vi "USBPT104Example.vi"() -> ()   [LabVIEW 2017]
uses:
  Instance           1 16Saved   USBPT104 .vi
  UsbPT104.dll
panel:
  out "UnitInfo fields":string[](array[string])=["Driver Version", "USB Version", "Hardware Version", "Variant Info", "Cal Date", "Kernal Driver Version"]
  out "error out":errorcluster={"status"=TRUE, "code"=5037, "source"="UsbPt104GetValue"}
  in  "error in (no error)":errorcluster
  out "UnitInfo":string[](array[string])
  in  "IP Address":string
  in  "Connection":bool
  out "CH4 Value":dbl(slide) max=10000.0 scale=-200.0..800.0
  out "CH3 Value":dbl(slide) max=10000.0 scale=-200.0..800.0
  out "CH2 Value":dbl(slide) max=10000.0 scale=-200.0..800.0
  in  "Update settings":bool
  in  "CH4 Measurement Type":i32(ring) items=["OFF", "PT100", "PT1000", "Resistance to 375 Ohms", "Resistance to 10 kOhms", "Differential to 115 mV", "Differential to 2500 mV", "Single-ended to 115 mV", "Single-ended to 2500 mV"]
  in  "CH4 Number of Wires":i16(ring)=4 items=["2"=2, "3"=3, "4"=4]
  in  "CH3 Measurement Type":i32(ring) items=["OFF", "PT100", "PT1000", "Resistance to 375 Ohms", "Resistance to 10 kOhms", "Differential to 115 mV", "Differential to 2500 mV", "Single-ended to 115 mV", "Single-ended to 2500 mV"]
  in  "CH3 Number of Wires":i16(ring)=4 items=["2"=2, "3"=3, "4"=4]
  in  "CH2 Measurement Type":i32(ring) items=["OFF", "PT100", "PT1000", "Resistance to 375 Ohms", "Resistance to 10 kOhms", "Differential to 115 mV", "Differential to 2500 mV", "Single-ended to 115 mV", "Single-ended to 2500 mV"]
  in  "CH2 Number of Wires":i16(ring)=4 items=["2"=2, "3"=3, "4"=4]
  in  "CH1 Number of Wires":i16(ring)=4 items=["2"=2, "3"=3, "4"=4]
  in  "CH1 Measurement Type":i32(ring)=1 items=["OFF", "PT100", "PT1000", "Resistance to 375 Ohms", "Resistance to 10 kOhms", "Differential to 115 mV", "Differential to 2500 mV", "Single-ended to 115 mV", "Single-ended to 2500 mV"]
  out "CH1 Value":dbl(slide) max=10000.0 scale=-200.0..800.0
  in  "Stop":bool
  # "USB"
  # "Ethernet"
  # "Channel 1"
  # "Channel 2"
  # "Channel 3"
  # "Channel 4"
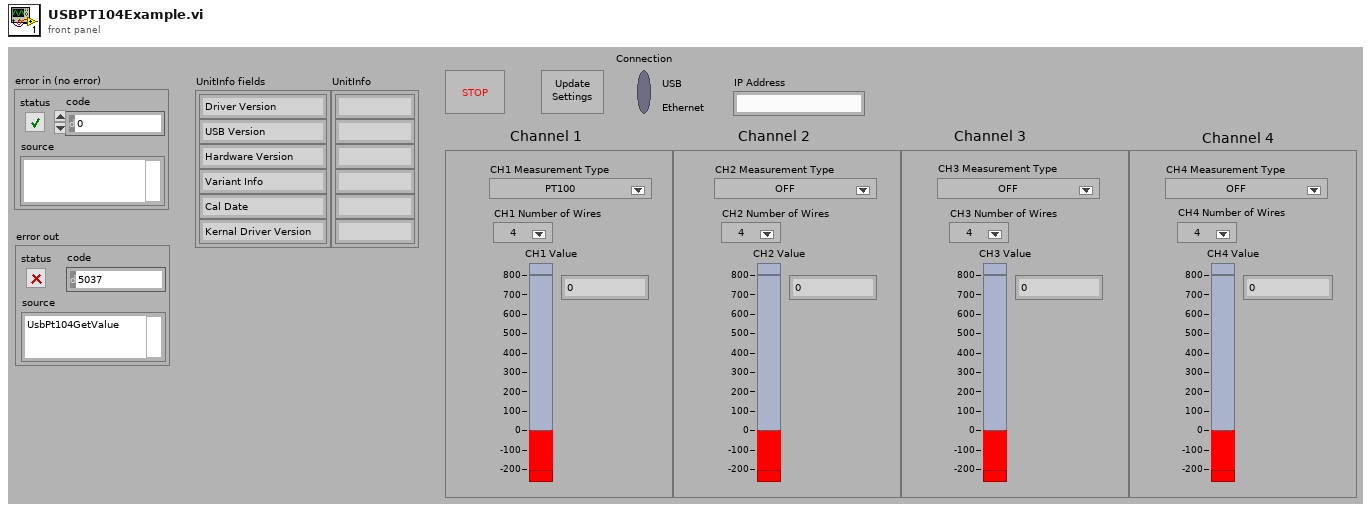
[diagram p1: front panel]
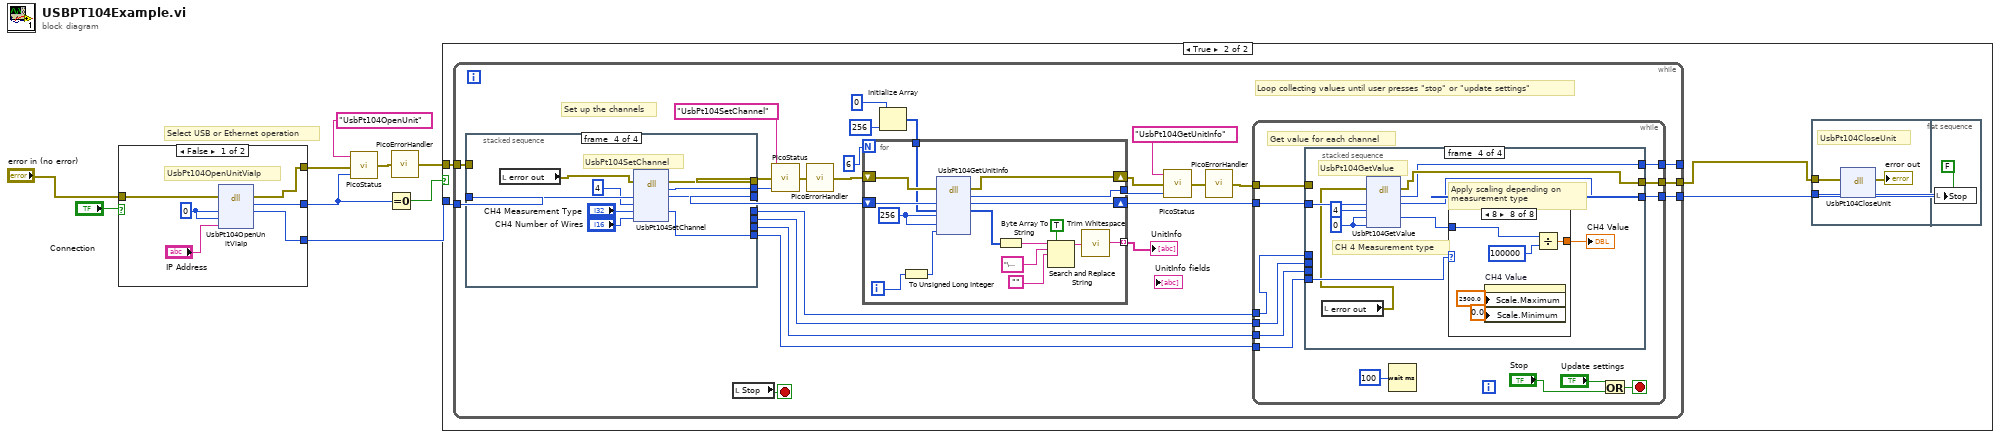
[diagram p0: block diagram]
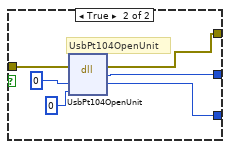
[diagram p2: hidden frame]
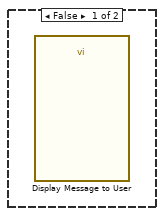
[diagram p3: hidden frame]
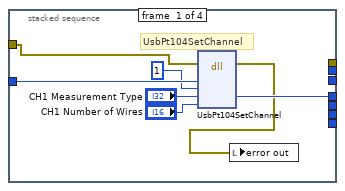
[diagram p4: hidden frame]
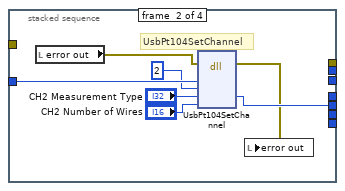
[diagram p5: hidden frame]
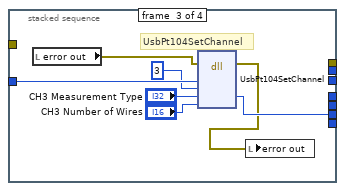
[diagram p6: hidden frame]
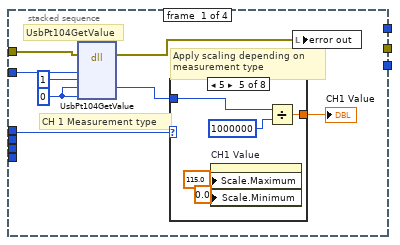
[diagram p7: hidden frame]
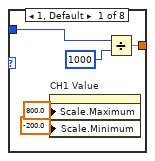
[diagram p8: hidden frame]
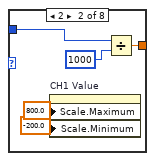
[diagram p9: hidden frame]
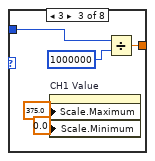
[diagram p10: hidden frame]
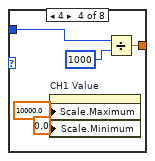
[diagram p11: hidden frame]
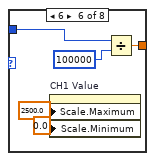
[diagram p12: hidden frame]
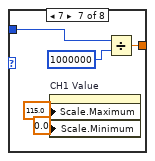
[diagram p13: hidden frame]
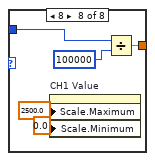
[diagram p14: hidden frame]
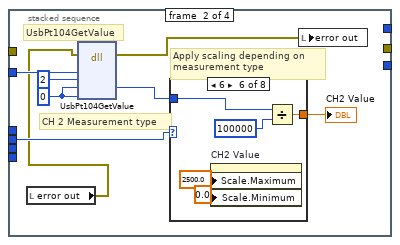
[diagram p15: hidden frame]
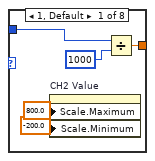
[diagram p16: hidden frame]
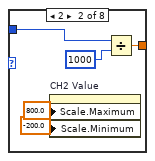
[diagram p17: hidden frame]
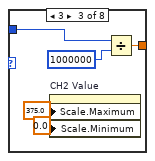
[diagram p18: hidden frame]
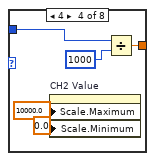
[diagram p19: hidden frame]
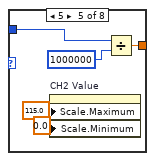
[diagram p20: hidden frame]
diagram:
  # "Select USB or Ethernet operation"
  n1 = case shown="False" "Connection" {
    tunnel: [w13 w21] -> w3
    tunnel: [w12 w19] -> w7
    tunnel: [w11 w20] -> w4
    tunnel: "error in (no error)" -> [w10 w16]
    frame False {
      w15 = i16 0 ("handle")
      # "UsbPt104OpenUnitViaIp"
      n2 = dll-call lib="UsbPT104.dll" fn="UsbPt104OpenUnitViaIp"(error in=w10, "handle"=w15, "serial"=w15, "IpAddress"="IP Address") -> (error out=w11:errorcluster, "Status"=w13:i32, "handle"=w12:i16)  [unwired: 4 in, 1 out]
    }
    frame True {
      # "UsbPt104OpenUnit"
      n3 = dll-call lib="UsbPT104.dll" fn="UsbPt104OpenUnit"(error in=w16, "handle"=i16 0, "serial"=0) -> (error out=w20:errorcluster, "Status"=w21:i32, "handle"=w19:i16)  [unwired: 3 in, 1 out]
    }
  }
  n4 = call "PicoStatus.vi"("PICO STATUS"=w3, "error in"=w4, "source"="UsbPt104OpenUnit") -> ("error out"=w6:errorcluster)
  n5 = Equal To 0?(x=w3) -> (x = 0?=w9:bool)
  n6 = call "PicoErrorHandler.vi"("error in"=w6) -> ("error out"=w2:errorcluster)
  n7 = case shown="True" w9 {
    tunnel: w7 -> [_ w24]
    tunnel: w2 -> [_ w23]
    frame False {
      n8 = call "Display Message to User"() -> ()  [unwired: 10 in, 2 out]
    }
    frame True {
      n9 = while {
        tunnel: w24 -> [w56]
        tunnel: [w55] -> w25
        tunnel: w23 -> [w32]
        tunnel: [w31] -> w22
        tunnel: [w30] -> _
        stop <- w54 stop-if-true
        # "Loop collecting values until user presses \"stop\" or \"update settings\""
        # "Set up the channels"
        n10 = stacked-sequence {
          tunnel: w56 -> [w79 w86 w93 w102]
          tunnel: [_ _ _ w98] -> w44
          tunnel: [w75 _ _ _] -> w53
          tunnel: [_ w82 _ _] -> w52
          tunnel: [_ _ w89 _] -> w51
          tunnel: [_ _ _ w97] -> w50
          tunnel: [_ _ _ w96] -> w46
          tunnel: [_ _ _ w95] -> w45
          tunnel: w32 -> [w74 _ _ _]
          frame #0 {
            # "UsbPt104SetChannel"
            n11 = dll-call lib="UsbPT104.dll" fn="UsbPt104SetChannel"(error in=w74, "handle"=w79, "channel"=1, "type"="CH1 Measurement Type", "noOfWires"="CH1 Number of Wires") -> (error out=w73:errorcluster, "type"=w75:i32)  [unwired: 6 in, 1 out]
            n12 = local write "error out"(w73) -> ()
          }
          frame #1 {
            # "UsbPt104SetChannel"
            n13 = local read "error out"() -> (w81:errorcluster)
            n14 = dll-call lib="UsbPT104.dll" fn="UsbPt104SetChannel"(error in=w81, "handle"=w86, "channel"=2, "type"="CH2 Measurement Type", "noOfWires"="CH2 Number of Wires") -> (error out=w80:errorcluster, "type"=w82:i32)  [unwired: 6 in, 1 out]
            n15 = local write "error out"(w80) -> ()
          }
          frame #2 {
            # "UsbPt104SetChannel"
            n16 = local read "error out"() -> (w88:errorcluster)
            n17 = dll-call lib="UsbPT104.dll" fn="UsbPt104SetChannel"(error in=w88, "handle"=w93, "channel"=3, "type"="CH3 Measurement Type", "noOfWires"="CH3 Number of Wires") -> (error out=w87:errorcluster, "type"=w89:i32)  [unwired: 6 in, 1 out]
            n18 = local write "error out"(w87) -> ()
          }
          frame #3 {
            # "UsbPt104SetChannel"
            n19 = local read "error out"() -> (w94:errorcluster)
            n20 = dll-call lib="UsbPT104.dll" fn="UsbPt104SetChannel"(error in=w94, "handle"=w102, "channel"=4, "type"="CH4 Measurement Type", "noOfWires"="CH4 Number of Wires") -> (error out=w96:errorcluster, "Status"=w95:i32, "handle"=w98:i16, "type"=w97:i32)  [unwired: 4 in, 1 out]
          }
        }
        n21 = local read "Stop"() -> (w54:bool)
        n22 = call "PicoStatus.vi"("PICO STATUS"=w45, "error in"=w46, "source"="UsbPt104SetChannel") -> ("error out"=w47:errorcluster)
        n23 = call "PicoErrorHandler.vi"("error in"=w47) -> ("error out"=w43:errorcluster)
        n24 = Initialize Array(u8 0 ("element"), 256 ("dimension size")) -> (w39:u8[])
        n25 = for {
          N: 6 -> [_]
          tunnel: [w59] -> w35 mode=indexing
          tunnel: [w64] -> w41
          tunnel: w39 -> [w62]
          shift-right: [w65] -> w42
          shift-left: w44 -> [w67]
          shift-right: [w63] -> w40
          shift-left: w43 -> [w66]
          i -> [w57]
          w68 = i16 256 ("stringLength")
          n26 = To Unsigned Long Integer(number=w57) -> (unsigned 32bit integer=w58:u32)
          n27 = dll-call lib="UsbPT104.dll" fn="UsbPt104GetUnitInfo"(error in=w66, "handle"=w67, "String"=w62, "StringLength"=w68, "requiredSize"=w68, "info"=w58) -> (error out=w63:errorcluster, "Status"=w64:i32, "handle"=w65:i16, "String"=w61:u8[])  [unwired: 5 in, 1 out]
          n28 = Byte Array To String(unsigned byte array=w61) -> (string=w60:string)
          n29 = Search and Replace String(replace all?=TRUE ("replace all? (F)"), input string=w60, search string="\u0000", replace string="") -> (result string=w69:string)  [unwired: 4 in, 3 out]
          n30 = call <vilib>:"Trim Whitespace.vi"("string"=w69) -> ("trimmed string"=w59:string)  [unwired: 1 in]
        }
        "UnitInfo" <- w35
        n31 = call "PicoStatus.vi"("PICO STATUS"=w41, "error in"=w40, "source"="UsbPt104GetUnitInfo") -> ("error out"=w34:errorcluster)
        n32 = call "PicoErrorHandler.vi"("error in"=w34) -> ("error out"=w33:errorcluster)
        n33 = while {
          tunnel: w42 -> [w106]
          tunnel: [w115] -> w55
          tunnel: w53 -> [w110]
          tunnel: w52 -> [w109]
          tunnel: w51 -> [w108]
          tunnel: w50 -> [w107]
          tunnel: w33 -> [w105]
          tunnel: [w104] -> w31
          tunnel: [w103] -> w30
          stop <- w113 stop-if-true
          # "Get value for each channel"
          n34 = stacked-sequence {
            tunnel: w106 -> [w123 w171 w219 w269]
            tunnel: [_ _ _ w266] -> w115
            tunnel: w110 -> [w118 _ _ _]
            tunnel: w109 -> [_ w166 _ _]
            tunnel: w108 -> [_ _ w214 _]
            tunnel: w107 -> [_ _ _ w263]
            tunnel: w105 -> [w117 _ _ _]
            tunnel: [_ _ _ w262] -> w104
            tunnel: [_ _ _ w260] -> w103
            frame #0 {
              w121 = 0 ("value")
              # "CH 1 Measurement type"
              # "Apply scaling depending on \nmeasurement type"
              # "UsbPt104GetValue"
              n35 = dll-call lib="UsbPT104.dll" fn="UsbPt104GetValue"(error in=w117, "handle"=w123, "channel"=1, "value"=w121, "filtered"=w121) -> (error out=w116:errorcluster, "value"=w120:i32)  [unwired: 6 in, 1 out]
              n36 = case shown="5" w118 {
                tunnel: w120 -> [w127 w132 w137 w142 w147 w152 w157 w162]
                tunnel: [w126 w131 w136 w141 w146 w151 w156 w161] -> w119
                frame 1, Default {
                  n37 = property on="CH1 Value" class="Slide (strict)"("Scale.Maximum"=800.0 ("Data Range:Maximum"), "Scale.Minimum"=-200.0 ("Scale.Range:Minimum")) -> ()  [unwired: 2 in, 2 out]
                  n38 = Divide(x=w127, y=1000) -> (x/y=w126:dbl)
                }
                frame 2 {
                  n39 = property on="CH1 Value" class="Slide (strict)"("Scale.Maximum"=800.0 ("Data Range:Maximum"), "Scale.Minimum"=-200.0 ("Scale.Range:Minimum")) -> ()  [unwired: 2 in, 2 out]
                  n40 = Divide(x=w132, y=1000) -> (x/y=w131:dbl)
                }
                frame 3 {
                  n41 = property on="CH1 Value" class="Slide (strict)"("Scale.Maximum"=375.0 ("Data Range:Maximum"), "Scale.Minimum"=0.0 ("Scale.Range:Minimum")) -> ()  [unwired: 2 in, 2 out]
                  n42 = Divide(x=w137, y=1000000) -> (x/y=w136:dbl)
                }
                frame 4 {
                  n43 = property on="CH1 Value" class="Slide (strict)"("Scale.Maximum"=10000.0 ("Data Range:Maximum"), "Scale.Minimum"=0.0 ("Scale.Range:Minimum")) -> ()  [unwired: 2 in, 2 out]
                  n44 = Divide(x=w142, y=1000) -> (x/y=w141:dbl)
                }
                frame 5 {
                  n45 = property on="CH1 Value" class="Slide (strict)"("Scale.Maximum"=115.0 ("Data Range:Maximum"), "Scale.Minimum"=0.0 ("Scale.Range:Minimum")) -> ()  [unwired: 2 in, 2 out]
                  n46 = Divide(x=w147, y=1000000) -> (x/y=w146:dbl)
                }
                frame 6 {
                  n47 = property on="CH1 Value" class="Slide (strict)"("Scale.Maximum"=2500.0 ("Data Range:Maximum"), "Scale.Minimum"=0.0 ("Scale.Range:Minimum")) -> ()  [unwired: 2 in, 2 out]
                  n48 = Divide(x=w152, y=100000) -> (x/y=w151:dbl)
                }
                frame 7 {
                  n49 = property on="CH1 Value" class="Slide (strict)"("Scale.Maximum"=115.0 ("Data Range:Maximum"), "Scale.Minimum"=0.0 ("Scale.Range:Minimum")) -> ()  [unwired: 2 in, 2 out]
                  n50 = Divide(x=w157, y=1000000) -> (x/y=w156:dbl)
                }
                frame 8 {
                  n51 = property on="CH1 Value" class="Slide (strict)"("Scale.Maximum"=2500.0 ("Data Range:Maximum"), "Scale.Minimum"=0.0 ("Scale.Range:Minimum")) -> ()  [unwired: 2 in, 2 out]
                  n52 = Divide(x=w162, y=100000) -> (x/y=w161:dbl)
                }
              }
              "CH1 Value" <- w119
              n53 = local write "error out"(w116) -> ()
            }
            frame #1 {
              w169 = 0 ("value")
              # "CH 2 Measurement type"
              # "Apply scaling depending on \nmeasurement type"
              # "UsbPt104GetValue"
              n54 = local read "error out"() -> (w164:errorcluster)
              n55 = dll-call lib="UsbPT104.dll" fn="UsbPt104GetValue"(error in=w164, "handle"=w171, "channel"=2, "value"=w169, "filtered"=w169) -> (error out=w165:errorcluster, "value"=w168:i32)  [unwired: 6 in, 1 out]
              n56 = case shown="6" w166 {
                tunnel: w168 -> [w175 w180 w185 w190 w195 w200 w205 w210]
                tunnel: [w174 w179 w184 w189 w194 w199 w204 w209] -> w167
                frame 1, Default {
                  n57 = property on="CH2 Value" class="Slide (strict)"("Scale.Maximum"=800.0 ("Data Range:Maximum"), "Scale.Minimum"=-200.0 ("Scale.Range:Minimum")) -> ()  [unwired: 2 in, 2 out]
                  n58 = Divide(x=w175, y=1000) -> (x/y=w174:dbl)
                }
                frame 2 {
                  n59 = property on="CH2 Value" class="Slide (strict)"("Scale.Maximum"=800.0 ("Data Range:Maximum"), "Scale.Minimum"=-200.0 ("Scale.Range:Minimum")) -> ()  [unwired: 2 in, 2 out]
                  n60 = Divide(x=w180, y=1000) -> (x/y=w179:dbl)
                }
                frame 3 {
                  n61 = property on="CH2 Value" class="Slide (strict)"("Scale.Maximum"=375.0 ("Data Range:Maximum"), "Scale.Minimum"=0.0 ("Scale.Range:Minimum")) -> ()  [unwired: 2 in, 2 out]
                  n62 = Divide(x=w185, y=1000000) -> (x/y=w184:dbl)
                }
                frame 4 {
                  n63 = property on="CH2 Value" class="Slide (strict)"("Scale.Maximum"=10000.0 ("Data Range:Maximum"), "Scale.Minimum"=0.0 ("Scale.Range:Minimum")) -> ()  [unwired: 2 in, 2 out]
                  n64 = Divide(x=w190, y=1000) -> (x/y=w189:dbl)
                }
                frame 5 {
                  n65 = property on="CH2 Value" class="Slide (strict)"("Scale.Maximum"=115.0 ("Data Range:Maximum"), "Scale.Minimum"=0.0 ("Scale.Range:Minimum")) -> ()  [unwired: 2 in, 2 out]
                  n66 = Divide(x=w195, y=1000000) -> (x/y=w194:dbl)
                }
                frame 6 {
                  n67 = property on="CH2 Value" class="Slide (strict)"("Scale.Maximum"=2500.0 ("Data Range:Maximum"), "Scale.Minimum"=0.0 ("Scale.Range:Minimum")) -> ()  [unwired: 2 in, 2 out]
                  n68 = Divide(x=w200, y=100000) -> (x/y=w199:dbl)
                }
                frame 7 {
                  n69 = property on="CH2 Value" class="Slide (strict)"("Scale.Maximum"=115.0 ("Data Range:Maximum"), "Scale.Minimum"=0.0 ("Scale.Range:Minimum")) -> ()  [unwired: 2 in, 2 out]
                  n70 = Divide(x=w205, y=1000000) -> (x/y=w204:dbl)
                }
                frame 8 {
                  n71 = property on="CH2 Value" class="Slide (strict)"("Scale.Maximum"=2500.0 ("Data Range:Maximum"), "Scale.Minimum"=0.0 ("Scale.Range:Minimum")) -> ()  [unwired: 2 in, 2 out]
                  n72 = Divide(x=w210, y=100000) -> (x/y=w209:dbl)
                }
              }
              "CH2 Value" <- w167
              n73 = local write "error out"(w165) -> ()
            }
            frame #2 {
              w217 = 0 ("value")
              # "CH 3 Measurement type"
              # "Apply scaling depending on \nmeasurement type"
              # "UsbPt104GetValue"
              n74 = local read "error out"() -> (w212:errorcluster)
              n75 = dll-call lib="UsbPT104.dll" fn="UsbPt104GetValue"(error in=w212, "handle"=w219, "channel"=3, "value"=w217, "filtered"=w217) -> (error out=w213:errorcluster, "value"=w216:i32)  [unwired: 6 in, 1 out]
              n76 = case shown="5" w214 {
                tunnel: w216 -> [w223 w228 w233 w238 w243 w248 w253 w258]
                tunnel: [w222 w227 w232 w237 w242 w247 w252 w257] -> w215
                frame 1, Default {
                  n77 = property on="CH3 Value" class="Slide (strict)"("Scale.Maximum"=800.0 ("Data Range:Maximum"), "Scale.Minimum"=-200.0 ("Scale.Range:Minimum")) -> ()  [unwired: 2 in, 2 out]
                  n78 = Divide(x=w223, y=1000) -> (x/y=w222:dbl)
                }
                frame 2 {
                  n79 = property on="CH3 Value" class="Slide (strict)"("Scale.Maximum"=800.0 ("Data Range:Maximum"), "Scale.Minimum"=-200.0 ("Scale.Range:Minimum")) -> ()  [unwired: 2 in, 2 out]
                  n80 = Divide(x=w228, y=1000) -> (x/y=w227:dbl)
                }
                frame 3 {
                  n81 = property on="CH3 Value" class="Slide (strict)"("Scale.Maximum"=375.0 ("Data Range:Maximum"), "Scale.Minimum"=0.0 ("Scale.Range:Minimum")) -> ()  [unwired: 2 in, 2 out]
                  n82 = Divide(x=w233, y=1000000) -> (x/y=w232:dbl)
                }
                frame 4 {
                  n83 = property on="CH3 Value" class="Slide (strict)"("Scale.Maximum"=10000.0 ("Data Range:Maximum"), "Scale.Minimum"=0.0 ("Scale.Range:Minimum")) -> ()  [unwired: 2 in, 2 out]
                  n84 = Divide(x=w238, y=1000) -> (x/y=w237:dbl)
                }
                frame 5 {
                  n85 = property on="CH3 Value" class="Slide (strict)"("Scale.Maximum"=115.0 ("Data Range:Maximum"), "Scale.Minimum"=0.0 ("Scale.Range:Minimum")) -> ()  [unwired: 2 in, 2 out]
                  n86 = Divide(x=w243, y=1000000) -> (x/y=w242:dbl)
                }
                frame 6 {
                  n87 = property on="CH3 Value" class="Slide (strict)"("Scale.Maximum"=2500.0 ("Data Range:Maximum"), "Scale.Minimum"=0.0 ("Scale.Range:Minimum")) -> ()  [unwired: 2 in, 2 out]
                  n88 = Divide(x=w248, y=100000) -> (x/y=w247:dbl)
                }
                frame 7 {
                  n89 = property on="CH3 Value" class="Slide (strict)"("Scale.Maximum"=115.0 ("Data Range:Maximum"), "Scale.Minimum"=0.0 ("Scale.Range:Minimum")) -> ()  [unwired: 2 in, 2 out]
                  n90 = Divide(x=w253, y=1000000) -> (x/y=w252:dbl)
                }
                frame 8 {
                  n91 = property on="CH3 Value" class="Slide (strict)"("Scale.Maximum"=2500.0 ("Data Range:Maximum"), "Scale.Minimum"=0.0 ("Scale.Range:Minimum")) -> ()  [unwired: 2 in, 2 out]
                  n92 = Divide(x=w258, y=100000) -> (x/y=w257:dbl)
                }
              }
              "CH3 Value" <- w215
              n93 = local write "error out"(w213) -> ()
            }
            frame #3 {
              w267 = 0 ("value")
              # "CH 4 Measurement type"
              # "Apply scaling depending on \nmeasurement type"
              # "UsbPt104GetValue"
              n94 = local read "error out"() -> (w261:errorcluster)
              n95 = dll-call lib="UsbPT104.dll" fn="UsbPt104GetValue"(error in=w261, "handle"=w269, "channel"=4, "value"=w267, "filtered"=w267) -> (error out=w262:errorcluster, "Status"=w260:i32, "handle"=w266:i16, "value"=w265:i32)  [unwired: 4 in, 1 out]
              n96 = case shown="8" w263 {
                tunnel: w265 -> [w273 w278 w283 w288 w293 w298 w303 w308]
                tunnel: [w272 w277 w282 w287 w292 w297 w302 w307] -> w264
                frame 1, Default {
                  n97 = property on="CH4 Value" class="Slide (strict)"("Scale.Maximum"=800.0 ("Data Range:Maximum"), "Scale.Minimum"=-200.0 ("Scale.Range:Minimum")) -> ()  [unwired: 2 in, 2 out]
                  n98 = Divide(x=w273, y=1000) -> (x/y=w272:dbl)
                }
                frame 2 {
                  n99 = property on="CH4 Value" class="Slide (strict)"("Scale.Maximum"=800.0 ("Data Range:Maximum"), "Scale.Minimum"=-200.0 ("Scale.Range:Minimum")) -> ()  [unwired: 2 in, 2 out]
                  n100 = Divide(x=w278, y=1000) -> (x/y=w277:dbl)
                }
                frame 3 {
                  n101 = property on="CH4 Value" class="Slide (strict)"("Scale.Maximum"=375.0 ("Data Range:Maximum"), "Scale.Minimum"=0.0 ("Scale.Range:Minimum")) -> ()  [unwired: 2 in, 2 out]
                  n102 = Divide(x=w283, y=1000000) -> (x/y=w282:dbl)
                }
                frame 4 {
                  n103 = property on="CH4 Value" class="Slide (strict)"("Scale.Maximum"=10000.0 ("Data Range:Maximum"), "Scale.Minimum"=0.0 ("Scale.Range:Minimum")) -> ()  [unwired: 2 in, 2 out]
                  n104 = Divide(x=w288, y=1000) -> (x/y=w287:dbl)
                }
                frame 5 {
                  n105 = property on="CH4 Value" class="Slide (strict)"("Scale.Maximum"=115.0 ("Data Range:Maximum"), "Scale.Minimum"=0.0 ("Scale.Range:Minimum")) -> ()  [unwired: 2 in, 2 out]
                  n106 = Divide(x=w293, y=1000000) -> (x/y=w292:dbl)
                }
                frame 6 {
                  n107 = property on="CH4 Value" class="Slide (strict)"("Scale.Maximum"=2500.0 ("Data Range:Maximum"), "Scale.Minimum"=0.0 ("Scale.Range:Minimum")) -> ()  [unwired: 2 in, 2 out]
                  n108 = Divide(x=w298, y=100000) -> (x/y=w297:dbl)
                }
                frame 7 {
                  n109 = property on="CH4 Value" class="Slide (strict)"("Scale.Maximum"=115.0 ("Data Range:Maximum"), "Scale.Minimum"=0.0 ("Scale.Range:Minimum")) -> ()  [unwired: 2 in, 2 out]
                  n110 = Divide(x=w303, y=1000000) -> (x/y=w302:dbl)
                }
                frame 8 {
                  n111 = property on="CH4 Value" class="Slide (strict)"("Scale.Maximum"=2500.0 ("Data Range:Maximum"), "Scale.Minimum"=0.0 ("Scale.Range:Minimum")) -> ()  [unwired: 2 in, 2 out]
                  n112 = Divide(x=w308, y=100000) -> (x/y=w307:dbl)
                }
              }
              "CH4 Value" <- w264
            }
          }
          n113 = Wait (ms)(milliseconds to wait=u32 100) -> ()  [unwired: 1 out]
          n114 = Or(x="Update settings", y="Stop") -> (x .or. y?=w113:bool)
        }
      }
      n115 = flat-sequence {
        tunnel: w25 -> [w28]
        tunnel: w22 -> [w27]
        frame #0 {
          # "UsbPt104CloseUnit"
          n116 = dll-call lib="UsbPT104.dll" fn="UsbPt104CloseUnit"(error in=w27, "handle"=w28) -> (error out=→"error out":errorcluster)  [unwired: 4 in, 1 out]
        }
        frame #1 {
          n117 = local write "Stop"(FALSE ("Stop")) -> ()
        }
      }
    }
  }
